vi "IND560 Stable Weigth Gross Not Equal Net.vi"(8 "Error In":errorcluster, 11 "read buffer":string) -> (0 "Error Out":errorcluster, 1 "IND560 Selector":T1, 2 "Gross Weight":dbl, 3 "Net Weight":dbl)   [LabVIEW 2016]
uses:
  Type Definitions/IND560 Data Output Selector.ctl
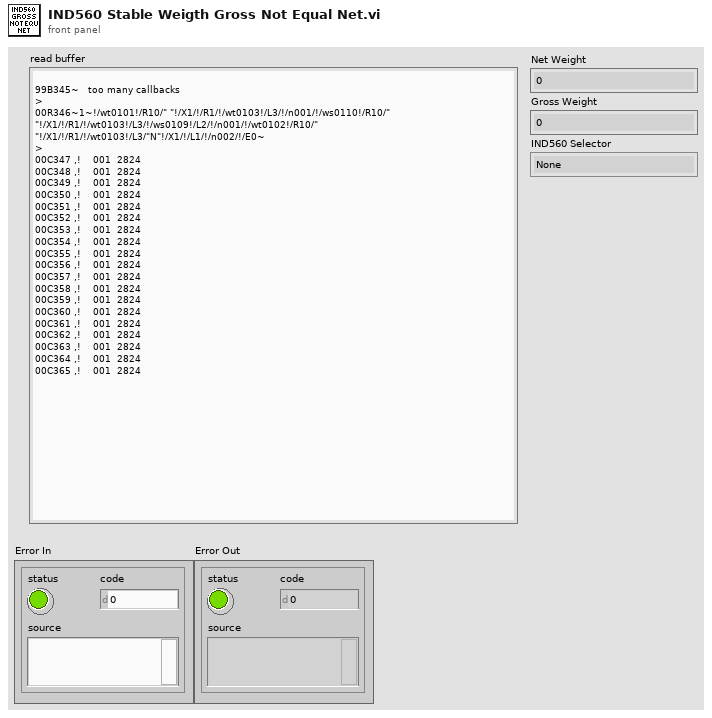
[diagram p1: front panel]
types:
  T1 = typedef "IND560 Data Output Selector.ctl" = enum16{"None", "Use Gross Not Equal Net", "Use Gross Equal Net", "Use Unstable Weights"}
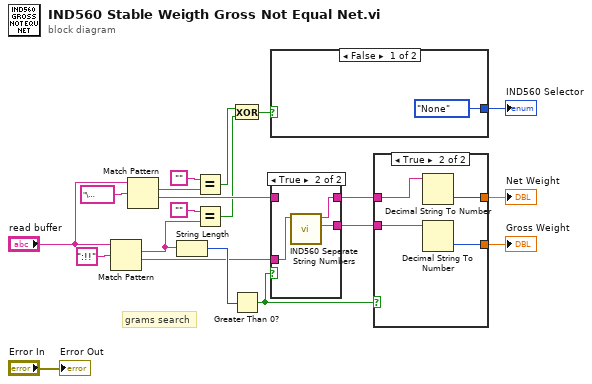
[diagram p0: block diagram]
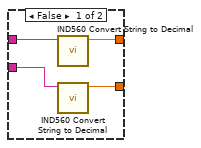
[diagram p2: hidden frame]
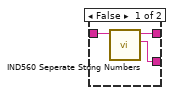
[diagram p3: hidden frame]
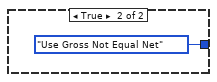
[diagram p4: hidden frame]
diagram:
  # "grams search"
  n1 = Match Pattern(string="read buffer", regular expression=":!!") -> (match substring=w3:string, after substring=w2:string)  [unwired: 1 in, 2 out]
  n2 = Match Pattern(string="read buffer", regular expression="\u0002,!    ") -> (match substring=w16:string, after substring=w19:string)  [unwired: 1 in, 2 out]
  n3 = String Length(string=w3) -> (length=w4:i32)
  n4 = Equal?(x="", y=w16) -> (x = y?=w7:bool)
  n5 = Equal?(x="", y=w3) -> (x = y?=w6:bool)
  n6 = Exclusive Or(1:w6, 2:w7) -> (0:w5:bool)
  n7 = Greater Than 0?(x=w4) -> (x > 0?=w1:bool)
  n8 = case shown="False" w5 {
    tunnel: [IND560_Data_Output_Selector."None" ("IND560 Selector") IND560_Data_Output_Selector."Use Gross Not Equal Net" ("IND560 Selector")] -> w14
    frame False {
    }
    frame True {
    }
  }
  "IND560 Selector" <- w14
  n9 = case shown="True" w1 {
    tunnel: w19 -> [w25 _]
    tunnel: [w23 w26] -> w12
    tunnel: [w24 w27] -> w11
    tunnel: w2 -> [_ w28]
    frame False {
      n10 = call "IND560 Seperate String Numbers.vi"("read buffer"=w25) -> ("Gross Weight"=w23:string, "Net Weight"=w24:string)  [unwired: 9 in]
    }
    frame True {
      n11 = call "IND560 Seperate String Numbers.vi"("read buffer"=w28) -> ("Gross Weight"=w26:string, "Net Weight"=w27:string)  [unwired: 9 in]
    }
  }
  n12 = case shown="True" w1 {
    tunnel: [w32 w33] -> w20
    tunnel: [w31 w34] -> w13
    tunnel: w12 -> [w30 w35]
    tunnel: w11 -> [w29 w36]
    frame False {
      n13 = call "IND560 Convert String to Decimal.vi"("read buffer"=w29) -> ("Weigth"=w32:dbl)  [unwired: 9 in, 1 out]
      n14 = call "IND560 Convert String to Decimal.vi"("read buffer"=w30) -> ("Weigth"=w31:dbl)  [unwired: 9 in, 1 out]
    }
    frame True {
      n15 = Decimal String To Number(string=w36) -> (number=w33:i32)  [unwired: 2 in, 1 out]
      n16 = Decimal String To Number(string=w35) -> (number=w34:i32)  [unwired: 2 in, 1 out]
    }
  }
  "Net Weight" <- w20
  "Gross Weight" <- w13
  "Error Out" <- "Error In"
